vi "lib Run Opendiff.vi"() -> ()   [LabVIEW 2011]
panel:
  out "error out":errorcluster
  in  "Cluster":T1
  out "Path 2":path
  out "Path":path
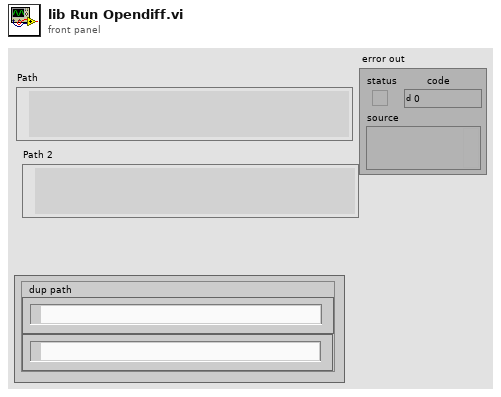
[diagram p1: front panel]
types:
  T1 = cluster{"dup path":path, "File Path Control":path}
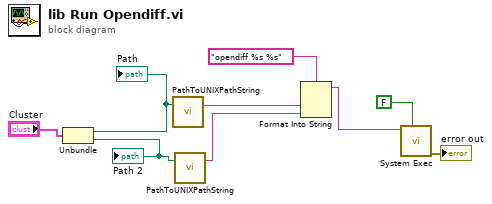
[diagram p0: block diagram]
diagram:
  n1 = Unbundle("Cluster") -> ("dup path"=w3:path, "File Path Control"=w2:path)
  "Path" <- w3
  "Path 2" <- w2
  n2 = call <vilib>:"PathToUNIXPathString.vi"("LV Path"=w3) -> ("UNIX Path"=w8:string)  [unwired: 1 in, 1 out]
  n3 = call <vilib>:"PathToUNIXPathString.vi"("LV Path"=w2) -> ("UNIX Path"=w7:string)  [unwired: 1 in, 1 out]
  n4 = Format Into String(format string="opendiff %s %s", w8, w7) -> (resulting string=w6:string)  [unwired: 2 in, 1 out]
  n5 = call <vilib>:"System Exec.vi"("wait until completion? (T)"=FALSE, "command line"=w6) -> ("error out"=→"error out":errorcluster)  [unwired: 6 in, 3 out]
